vi "Display UI.vi"(8 "error in (no error)":errorcluster, 11 "Configuration in":refnum<class "Configuration.lvclass">) -> (0 "error out":errorcluster, 3 "Configuration out":refnum<class "Configuration.lvclass">)   [LabVIEW 2016, in "Configuration.lvlib" / "Configuration.lvclass"]
doc: "This method displays the actor core of the leaf in the class hierarchy. This ensures that only the most specific definition of a UI is displayed, and no ancestors are seen by the user"
uses:
  <userlib>/Configuration Dialog Actor/Configuration.lvclass
  <userlib>/Configuration Dialog Actor/Configuration.lvclass/Configuration.ctl
  <userlib>/Configuration Dialog Actor/Accessors/Write VI to Display.vi
  <userlib>/Configuration Dialog Actor/Accessors/Read VI to Display.vi
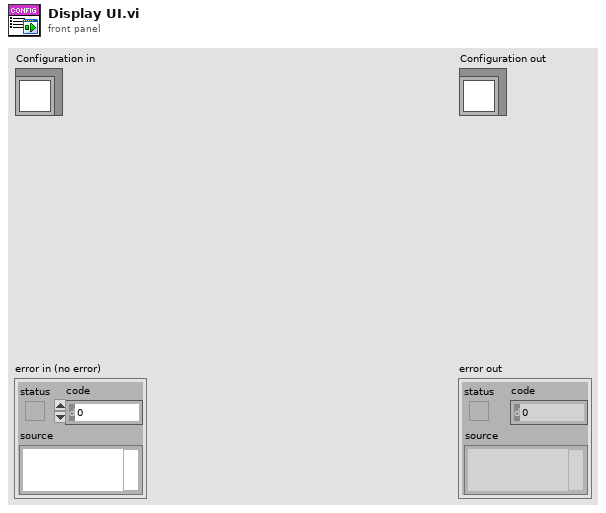
[diagram p1: front panel]
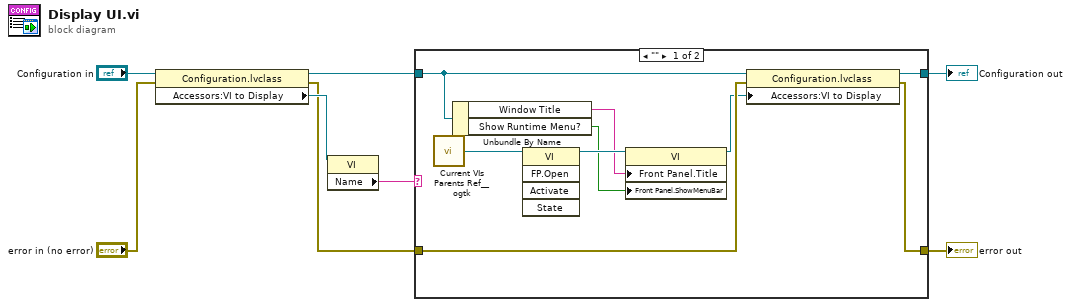
[diagram p0: block diagram]
diagram:
  n1 = property class="Configuration.lvclass"(reference="Configuration in", error in="error in (no error)") -> (reference out=w6:refnum<class "Configuration.lvclass">, error out=w2:errorcluster, "Accessors:VI to Display"=w5:refnum<vi>)
  n2 = property class="VI"(reference=w5) -> ("Name"=w4:string)  [unwired: 1 in, 2 out]
  n3 = case shown="\"\"" w4 {
    tunnel: [w16 w19] -> w7
    tunnel: w6 -> [w11 w19]
    tunnel: w2 -> [w14 w18]
    tunnel: [w13 w18] -> w1
    frame "" {
      n4 = call <userlib>:"Current VIs Parents Ref__ogtk.vi"() -> ("Calling VI's Reference"=w17:refnum<vi>)  [unwired: 2 in]
      n5 = Unbundle By Name(w11) -> ("Window Title"=w10:string, "Show Runtime Menu?"=w9:bool)
      n6 = invoke class="VI" method="FP.Open"(reference=w17) -> (reference out=w15:refnum<vi>)  [unwired: 4 in, 4 out]
      n7 = property class="VI"(reference=w15, "Front Panel.Title"=w10, "Front Panel.ShowMenuBar"=w9) -> (reference out=w12:refnum<vi>)  [unwired: 1 in, 1 out]
      n8 = property class="Configuration.lvclass"(reference=w11, error in=w14, "Accessors:VI to Display"=w12) -> (reference out=w16:refnum<class "Configuration.lvclass">, error out=w13:errorcluster)
    }
    frame Default {
    }
  }
  "error out" <- w1
  "Configuration out" <- w7
